vi "Write Config File.vi"(8 "error in (no error)":errorcluster, 11 "[C] User Management in":refnum<class "[C] User Management.lvclass">) -> (0 "error out":errorcluster, 3 "[C] User Management out":refnum<class "[C] User Management.lvclass">)   [LabVIEW 2020]
uses:
  <vilib>/Utility/config.llb/NI_LVConfig.lvlib
  <userlib>/_OpenG.lib/variantconfig/variantconfig.llb/openg_variant_configuration_file.lvlib
  [C] User Management.lvclass
  C:/Program Files (x86)/National Instruments/LabVIEW 2020/vi.lib/ActorFramework/Actor/Actor.lvclass
  D:/03 GitHub/LabVIEW-User-Management/[C] User Management/[C] User Management/[C] User Management.lvclass
  D:/03 GitHub/LabVIEW-User-Management/[V] Login/INF of [V] Login/INF of [V] Login.lvclass
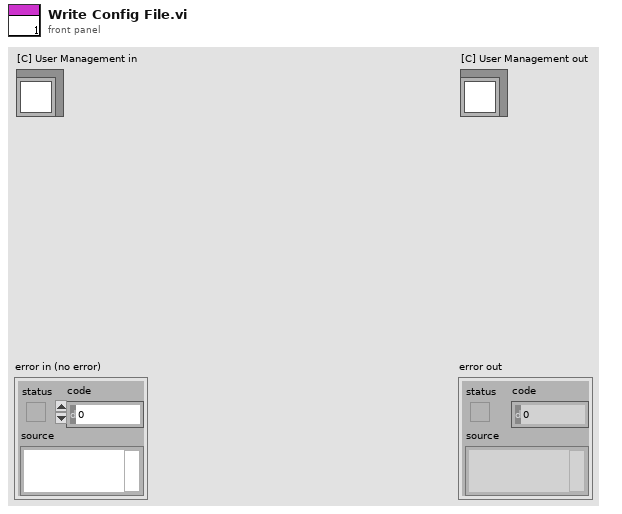
[diagram p1: front panel]
types:
  T1 = typedef "NI_LVConfig.lvlib/Config Data RefNum.ctl" = refnum<k1>
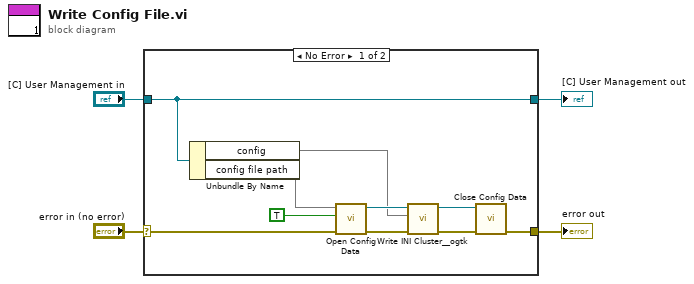
[diagram p0: block diagram]
diagram:
  n1 = case shown="No Error" "error in (no error)" {
    selector: "error in (no error)" -> [w14 w16]
    tunnel: [w5 w16] -> w3
    tunnel: [w6 w15] -> w1
    tunnel: "[C] User Management in" -> [w6 w15]
    frame No Error {
      n2 = Unbundle By Name(w6) -> ("config"=w9, "config file path"=w13)
      n3 = call <vilib>:"Open Config Data.vi"("error in (no error)"=w14, "create file if necessary (T)"=TRUE, "configuration file path"=w13) -> ("error out"=w11:errorcluster, "refnum"=w10:T1)  [unwired: 6 in, 1 out]
      n4 = call <userlib>:"Write INI Cluster__ogtk.vi"("error in (no error)"=w11, "INI Fomatted Cluster"=w9, "refnum"=w10) -> ("error out"=w8:errorcluster, "dup refnum"=w7:T1)  [unwired: 7 in]
      n5 = call <vilib>:"Close Config Data.vi"("error in (no error)"=w8, "refnum"=w7) -> ("error out"=w5:errorcluster)  [unwired: 8 in, 1 out]
    }
    frame Error {
    }
  }
  "error out" <- w3
  "[C] User Management out" <- w1
